vi "Get Transfer Configuration.vi"(8 "error in (no error)":errorcluster, 11 "Component Configuration in":refnum<class "Default Buffer Converter Configurations.lvclass">) -> (0 "error out":errorcluster, 1 "Tx Transfer Configuration":refnum<class "Configuration.lvclass">, 2 "Rx Transfer Configuration":refnum<class "Configuration.lvclass">, 3 "Component Configuration out":refnum<class "Default Buffer Converter Configurations.lvclass">)   [LabVIEW 2019, in "DSF Core.lvlib" / "Default Buffer Converter Configurations.lvclass"]
uses:
  Default Buffer Converter Configurations.lvclass
  Classes/Configuration/Configuration.lvclass
  Default Buffer Converter Transfer Configuration.lvclass
  C:/Dev/GitHub/niveristand-data-sharing-framework-custom-device/Core/Classes/Configuration/Configuration.lvclass
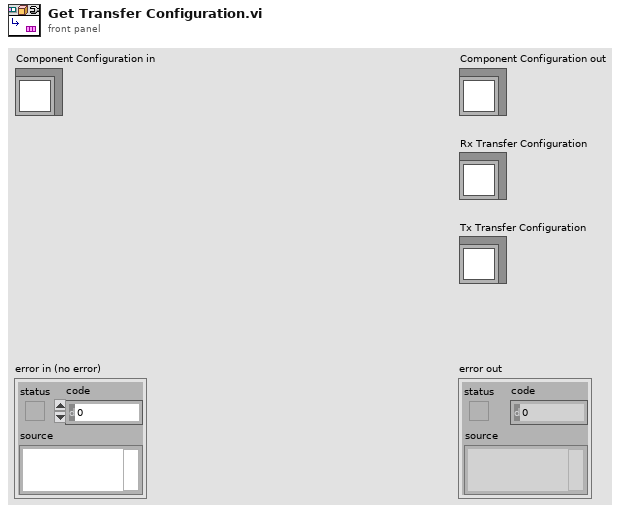
[diagram p1: front panel]
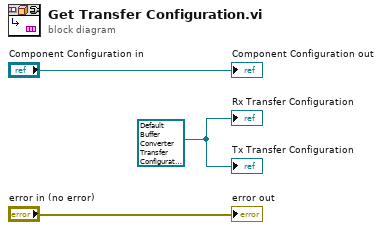
[diagram p0: block diagram]
diagram:
  w1 = refnum<class "Default Buffer Converter Transfer Configuration.lvclass"> refnum ("DSF Core.lvlib:DSF Buffer Converter Transfer Configuration.lvclass")
  "error out" <- "error in (no error)"
  "Component Configuration out" <- "Component Configuration in"
  "Rx Transfer Configuration" <- w1
  "Tx Transfer Configuration" <- w1
